vi "LabS3_Probe1.vi"() -> ()   [LabVIEW 2012]
panel:
  out "bf":dbl
  out "X1":dbl[](array[numeric])
  out "X2":dbl[](array[numeric])
  out "XY Graph":cluster{"Y":dbl[], "Y":dbl[]}[](graph)
  in  "h":dbl
  in  "ti":dbl
  in  "tf":dbl
  out "wf":dbl[](array[numeric])
  out "w":dbl[](array[numeric])
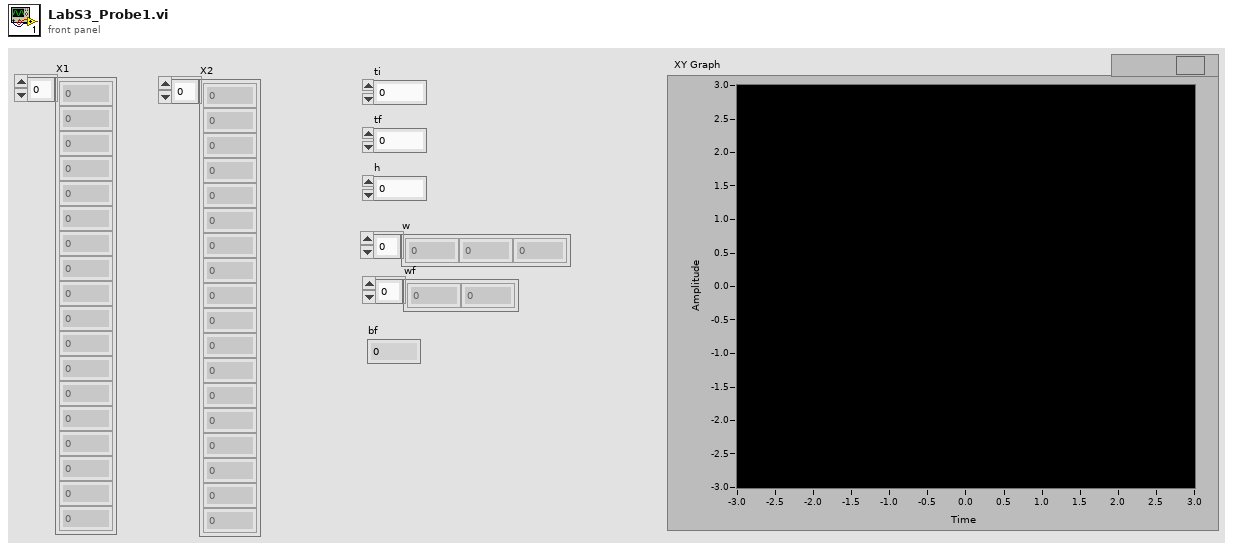
[diagram p1: front panel]
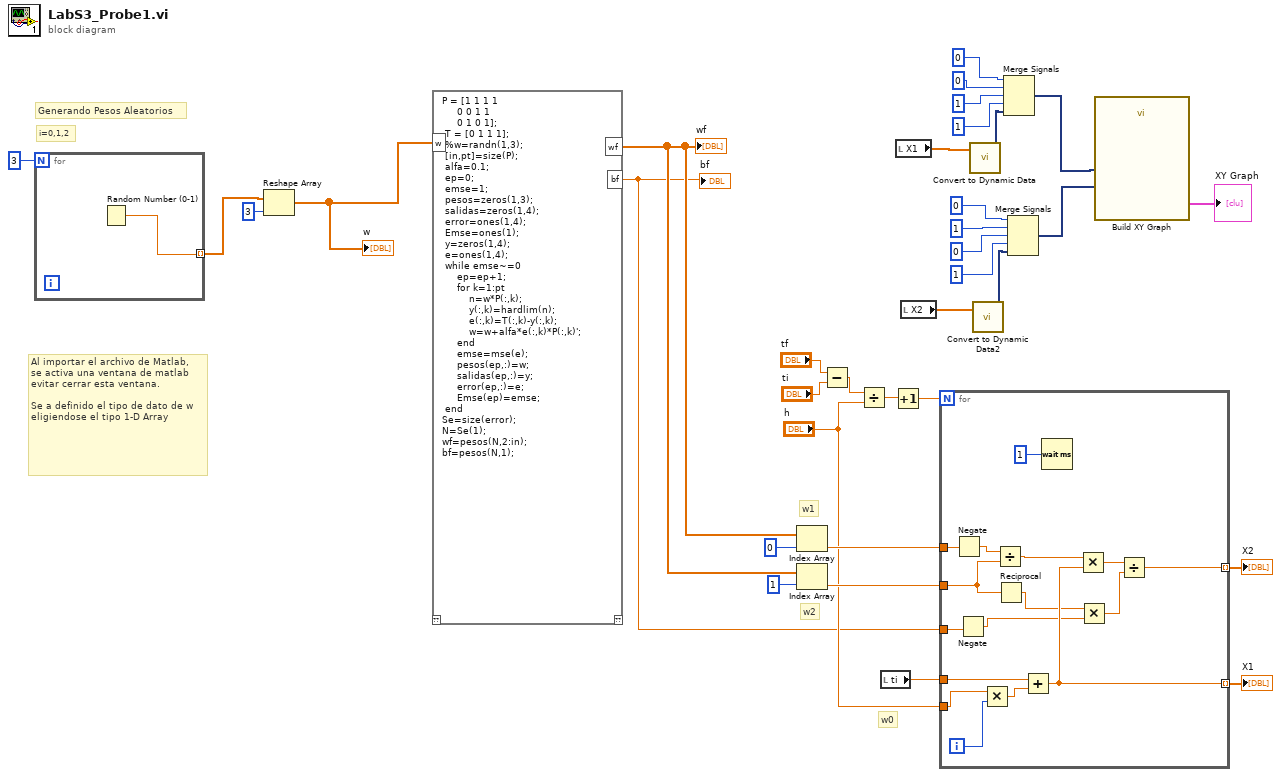
[diagram p0: block diagram]
diagram:
  # "w0"
  # "w1"
  # "w2"
  # "Al importar el archivo de Matlab,\nse activa una ventana de matlab\nevitar cerrar esta ventana.\n\nSe a definido el tipo de dato de w\neligiendose el tipo 1-D Array"
  # "Generando Pesos Aleatorios"
  # "i=0,1,2"
  n1 = for {
    N: 3 -> [_]
    tunnel: [w35] -> w33 mode=indexing
    n2 = Random Number (0-1)() -> (number: 0 to 1=w35:dbl)
  }
  n3 = Reshape Array(w33, 3 ("dimension size")) -> (w31:dbl[])
  "w" <- w31
  n4 = script code="P = [1 1 1 1\n     0 0 1 1\n     0 1 0 1];\n T = [0 1 1 1];\n %w=randn(1,3);\n [in,pt]=size(P);\n alfa=0.1; \n ep=0; \n emse=1;\n pesos=zeros(1,3);\n salidas=zeros(1,4);\n error=ones(1,4);\n Emse=ones(1);\n y=zeros(1,4);\n e=ones(1,4);\n while emse~=0\n     ep=ep+1;\n     for k=1:pt\n         n=w*P(:,k);\n         y(:,k)=hardlim(n);\n         e(:,k)=T(:,k)-y(:,k);\n         w=w+alfa*e(:,k)*P(:,k)';\n     end\n     emse=mse(e);\n     pesos(ep,:)=w;\n     salidas(ep,:)=y;\n     error(ep,:)=e;\n     Emse(ep)=emse;\n end\nSe=size(error);\nN=Se(1);\nwf=pesos(N,2:in);\nbf=pesos(N,1);"("w"=w31) -> ("wf"=w23:dbl[], "bf"=w1:dbl)  [unwired: 1 in, 1 out]
  "wf" <- w23
  "bf" <- w1
  n5 = Index Array(array=w23, index=0 ("dimension size")) -> (element=w21:dbl)
  n6 = Index Array(array=w23, index=1 ("dimension size")) -> (element=w22:dbl)
  n7 = Subtract(x="tf", y="ti") -> (x-y=w28:dbl)
  n8 = Divide(x=w28, y="h") -> (x/y=w27:dbl)
  n9 = local read "ti"() -> (w20:dbl)
  n10 = Increment(x=w27) -> (x+1=w26:dbl)
  n11 = local read "X1"() -> (w2:dbl[])
  n12 = local read "X2"() -> (w3:dbl[])
  n13 = for {
    N: w26 -> [_]
    tunnel: "h" -> [w51]
    tunnel: w22 -> [w40]
    tunnel: w21 -> [w46]
    tunnel: w20 -> [w48]
    tunnel: [w43] -> w4 mode=indexing
    tunnel: [w41] -> w5 mode=indexing
    tunnel: w1 -> [w36]
    i -> [w50]
    n14 = Negate(x=w46) -> (-x=w45:dbl)
    n15 = Negate(x=w36) -> (-x=w38:dbl)
    n16 = Multiply(x=w51, y=w50) -> (x*y=w49:dbl)
    n17 = Divide(x=w45, y=w40) -> (x/y=w44:dbl)
    n18 = Reciprocal(x=w40) -> (1/x=w39:dbl)
    n19 = Add(x=w48, y=w49) -> (x+y=w43:dbl)
    n20 = Wait (ms)(milliseconds to wait=u32 1) -> ()  [unwired: 1 out]
    n21 = Multiply(x=w44, y=w43) -> (x*y=w42:dbl)
    n22 = Multiply(x=w39, y=w38) -> (x*y=w37:dbl)
    n23 = Divide(x=w42, y=w37) -> (x/y=w41:dbl)
  }
  "X2" <- w5
  "X1" <- w4
  n24 = call "Convert to Dynamic Data"("Array"=w2) -> ("Dynamic Data Type"=w7:dynamicdata)  [unwired: 3 in]
  n25 = call "Convert to Dynamic Data2"("Array"=w3) -> ("Dynamic Data Type"=w6:dynamicdata)  [unwired: 3 in]
  n26 = Merge Signals(0, 0, 1, 1, w7) -> (w16:dynamicdata)
  n27 = Merge Signals(0, 1, 0, 1, w6) -> (w17:dynamicdata)
  n28 = call "Build XY Graph"("Y Input"=w17, "X Input"=w16) -> ("XY Graph"=→"XY Graph":cluster{"Y":dbl[], "Y":dbl[]}[])  [unwired: 3 in, 6 out]
